vi "Write 1D Array.vi"(8 "error in (no error)":errorcluster, 10 "1D Array":dbl[](array[numeric]), 11 "Data1D in":refnum<class "Data1D.lvclass">) -> (0 "error out":errorcluster, 3 "Data1D out":refnum<class "Data1D.lvclass">)   [LabVIEW 2014, in "Data1D.lvclass"]
uses:
  Data1D.lvclass
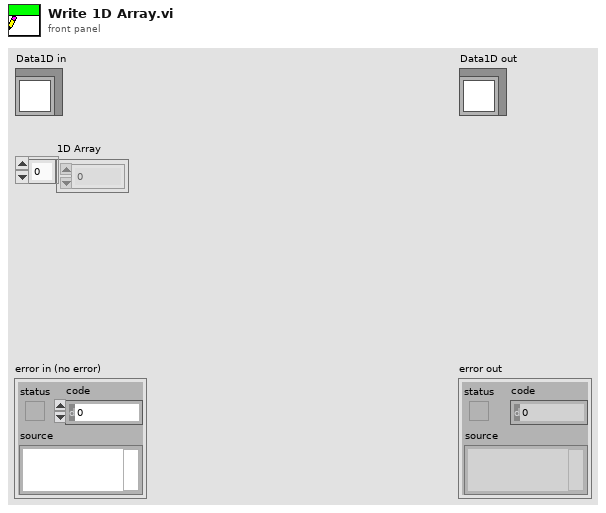
[diagram p1: front panel]
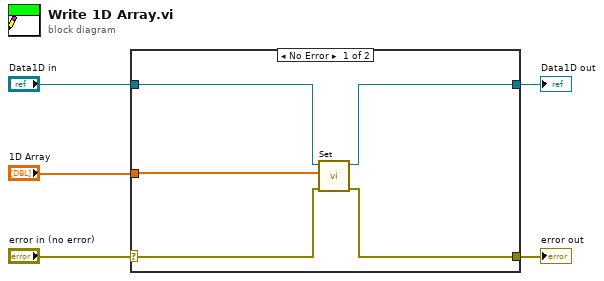
[diagram p0: block diagram]
diagram:
  n1 = case shown="No Error" "error in (no error)" {
    selector: "error in (no error)" -> [w7 w11]
    tunnel: [w6 w11] -> w4
    tunnel: [w8 w12] -> w2
    tunnel: "Data1D in" -> [w9 w12]
    tunnel: "1D Array" -> [w10 _]
    frame No Error {
      n2 = call-dynamic "Set.vi"("error in (no error)"=w7, "Data"=w10, "AbstractData in"=w9) -> ("error out"=w6:errorcluster, "AbstractData out"=w8:refnum<class "Data1D.lvclass">)  [unwired: 7 in]
    }
    frame Error {
    }
  }
  "error out" <- w4
  "Data1D out" <- w2
